vi "TIRF_ButtonHelper.vi"(10 "Stop":bool, 11 "Button Ref":refnum<vi>) -> ()   [LabVIEW 2010]
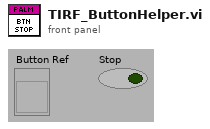
[diagram p1: front panel]
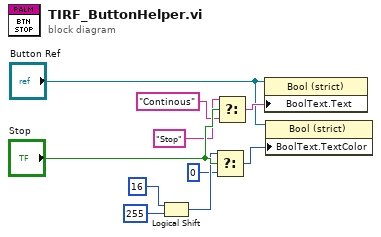
[diagram p0: block diagram]
diagram:
  n1 = Logical Shift(y=u32 16 ("x"), x=u32 255 ("Boolean Text.Text Colors:Text Color")) -> (x << y=w8:u32)
  n2 = Select(t=w8, s="Stop", f=u32 0) -> (s? t:f=w9:u32)
  n3 = Select(t="Stop" ("Boolean Text.Text"), s="Stop", f="Continous" ("Boolean Text.Text")) -> (s? t:f=w6:string)
  n4 = property on="Property Node" class="Bool (strict)"(reference="Button Ref", "BoolText.Text"=w6) -> ()  [unwired: 1 in, 2 out]
  n5 = property on="Property Node" class="Bool (strict)"(reference="Button Ref", "BoolText.TextColor"=w9) -> ()  [unwired: 1 in, 2 out]
